vi "Get ColumnsName.vi"(8 "error in (no error)":errorcluster, 10 "TableName":string, 11 "SQLite_API in":refnum<class "SQLite_API.lvclass">) -> (0 "error out":errorcluster, 1 "column information":T2(array[cluster]), 2 "Table_ColunmsList":string[](array[string]), 3 "SQLite_API out":refnum<class "SQLite_API.lvclass">)   [LabVIEW 2021, in "SQLite_API.lvclass"]
uses:
  <userlib>/John_Lib/DataBase/SQLite_API/SQLite_API.lvclass
  <userlib>/John_Lib/DataBase/SQLite_API/SQLite_API.lvclass/SQLite_API.ctl
  <vilib>/drjdpowell/SQLite Library/SQL Connection/Connection.lvclass
  <vilib>/drjdpowell/SQLite Library/SQL Statement/SQL Statement.lvclass
  <vilib>/addons/database/Auxilliary.llb/DB Tools DataTypes.ctl
  <vilib>/addons/database/NI_Database_API.lvlib
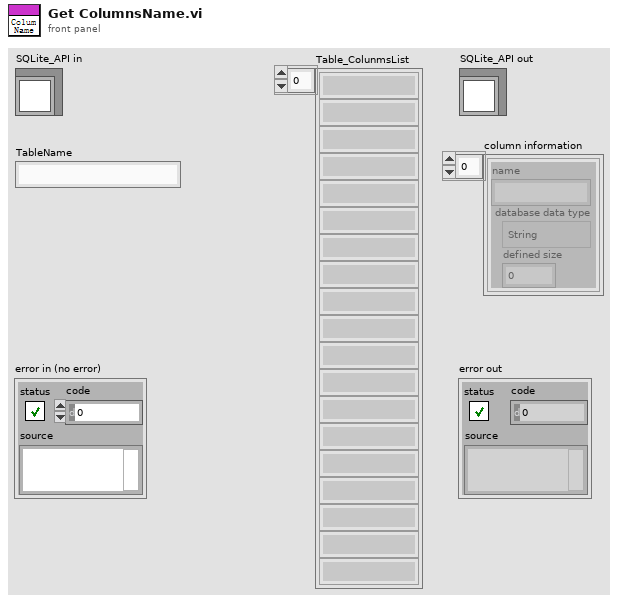
[diagram p1: front panel]
types:
  T1 = typedef "NI_Database_API.lvlib/DB Tools DataTypes.ctl" = enum16{"String", "Long (I32)", "Single (SGL)", "Double (DBL)", "Date/Time", "Binary"}
  T2 = cluster{"name":string, "database data type":T1, "defined size":i32}[]
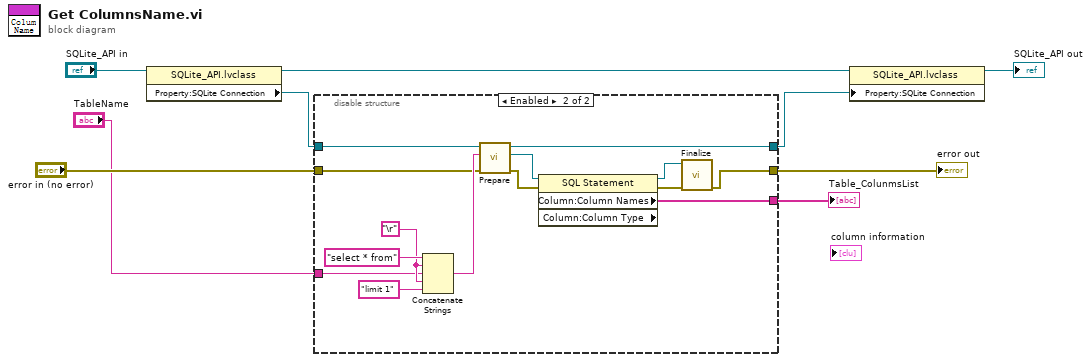
[diagram p0: block diagram]
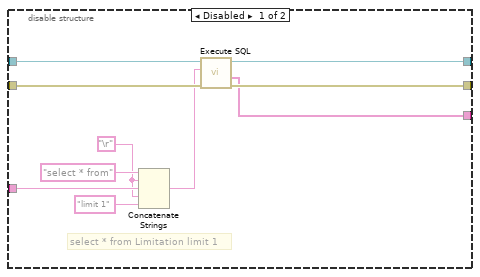
[diagram p2: hidden frame]
diagram:
  n1 = property class="SQLite_API.lvclass"(reference="SQLite_API in") -> (reference out=w8:refnum<class "SQLite_API.lvclass">, "Property:SQLite Connection"=w7:refnum<class "Connection.lvclass">)  [unwired: 1 in, 1 out]
  n2 = disable-structure shown="Enabled" {
    disable-tunnel: w7 -> [w19 w33]
    disable-tunnel: [w18 w26] -> w2
    disable-tunnel: "error in (no error)" -> [w17 w27]
    disable-tunnel: [w16 w20] -> w5
    disable-tunnel: [w15 w24] -> w1
    disable-tunnel: "TableName" -> [w13 w29]
    frame Disabled {
      w12 = "\r"
      # "select * from Limitation limit 1"
      n3 = Concatenate Strings("select * from" ("string"), w12, w13, w12, "limit 1" ("string")) -> (w10:string)
      n4 = call <vilib>:"Execute SQL.vi"("error in (no error)"=w17, "SQL"=w10, "SQLite Connection in"=w19) -> ("error out"=w16:errorcluster, "Column Names"=w15:string[], "SQLite Connection"=w18:refnum<class "Connection.lvclass">)  [unwired: 5 in, 1 out]
    }
    frame Enabled {
      w31 = "\r"
      n5 = Concatenate Strings("select * from" ("string"), w31, w29, w31, "limit 1" ("string")) -> (w28:string)
      n6 = call <vilib>:"Prepare.vi"("error in (no error)"=w27, "SQL"=w28, "SQLite Connection in"=w33) -> ("error out"=w23:errorcluster, "SQL Statement"=w25:refnum<class "SQL Statement.lvclass">, "SQLite Connection"=w26:refnum<class "Connection.lvclass">)  [unwired: 4 in, 2 out]
      n7 = property class="SQL Statement" props=["Column:Column Names", "Column:Column Type"](reference=w25, error in=w23) -> (reference out=w22:refnum<class "SQL Statement.lvclass">, error out=w21:errorcluster, "Column:Column Names"=w24:string[])  [unwired: 1 out]
      n8 = call <vilib>:"Finalize.vi"("error in (no error)"=w21, "SQL Statement in"=w22) -> ("error out"=w20:errorcluster)  [unwired: 9 in]
    }
  }
  "error out" <- w5
  "Table_ColunmsList" <- w1
  n9 = property class="SQLite_API.lvclass"(reference=w8, "Property:SQLite Connection"=w2) -> (reference out=→"SQLite_API out":refnum<class "SQLite_API.lvclass">)  [unwired: 1 in, 1 out]
